vi "Line Configuration Dialog.vi"(8 "error in":errorcluster, 9 "engine configuration in":refnum<class "engine configuration.lvclass">, 10 "tag bus configurable plugin module configuration":refnum<class "SQLite configuration.lvclass">, 11 "Line":T3) -> (0 "error out":errorcluster, 1 "success":bool, 2 "changed":bool, 3 "Mappings out":T2)   [LabVIEW 2014, in "SQLite editor node.lvclass"]
doc: "A dialog for allowing a user to specify the values of a new line."
uses:
  SQLite editor node.lvclass
  module/configuration/Line.ctl
  <vilib>/NI/Tag Bus Module Framework/channel/TBM channel.lvclass
  Mappings.ctl
  Map.ctl
  permissions.ctl
  <vilib>/NI/Module Execution Interface/Engine Configuration/engine configuration.lvclass
  module/configuration/SQLite configuration.lvclass
  <vilib>/NI/Tag Bus Module Framework/channel/TBM channel.lvclass/TBM channel.ctl
  <vilib>/NI/Tag Bus/tag/tag descriptor.lvclass/tag descriptor.ctl
  <vilib>/NI/Configuration Framework/serializable configuration/NISE_CEF_serializable configuration.lvclass/NISE_CEF_serializable configuration.ctl
  <vilib>/NI/Tag Bus/tag/write tag name.vi
  <vilib>/NI/Tag Bus/tag/write data type.vi
  <vilib>/NI/Tag Bus Module Framework/channel/Write channel classification.vi
  <vilib>/NI/Configuration Framework/serializable configuration/Read UID.vi
  <vilib>/NI/Tag Bus Module Framework/channel/Read channel classification.vi
  <vilib>/NI/Tag Bus/tag/read data type.vi
  <vilib>/Utility/LVClass/Get LV Class Name.vi
  <vilib>/NI/Configuration Framework/error generator/NISE_error generator.vi
  <vilib>/NI/Tag Bus/tag/tag descriptor.lvclass
  <vilib>/NI/DCAF UI Toolkit/Controls/DCAF UI Elements.lvlib
panel:
  out "errors":string
  in  "Access Type":T1
  in  "Tag":i32(listbox)
  in  "Data Type":i32(listbox)
  in  "Channel Name":string
  in  "cancel":bool
  in  "ok":bool
  # "#CodeRecommended Add implementation details here. For example, a shared variable URL."
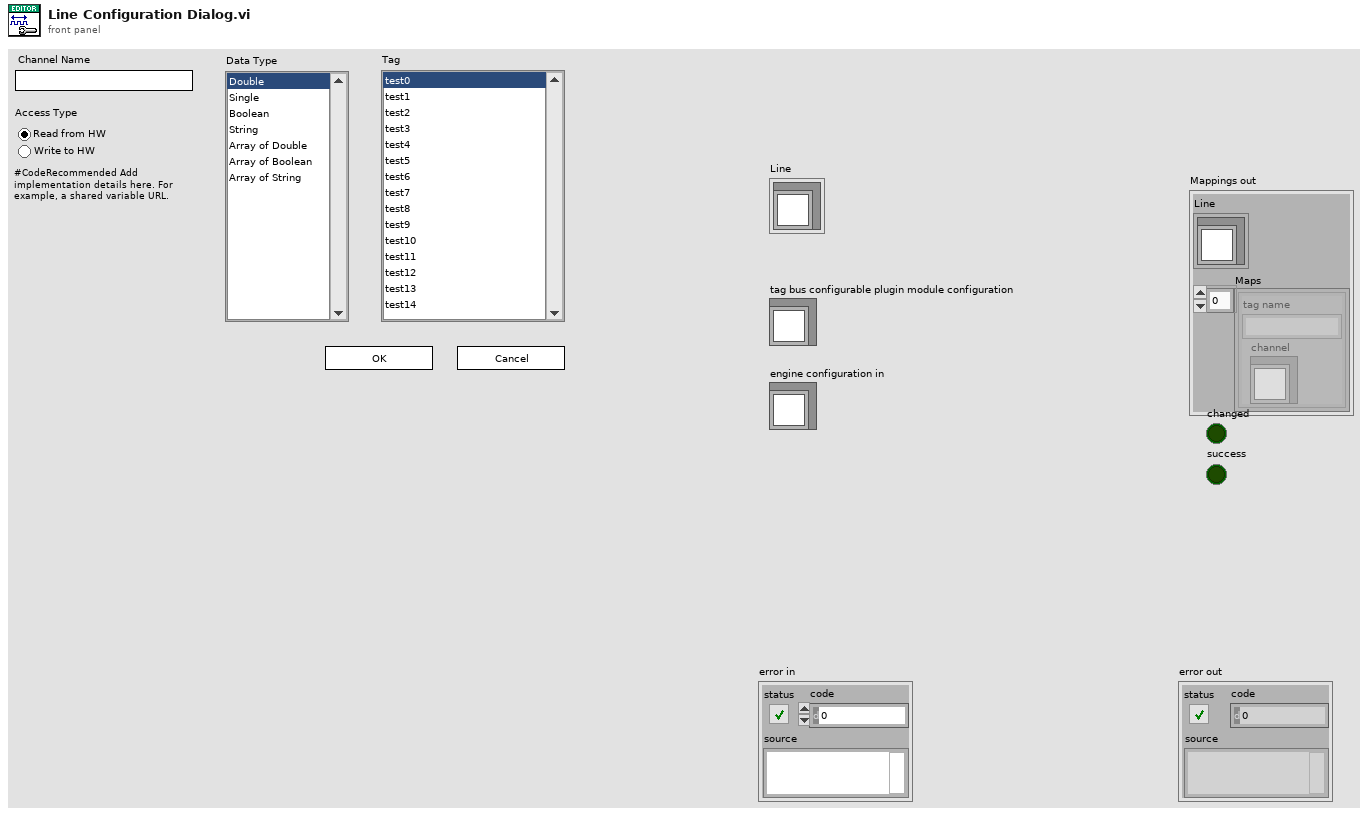
[diagram p1: front panel]
types:
  T1 = typedef "SQLite editor node.lvclass/permissions.ctl" = enum32{"Read from HW", "Write to HW"}
  T2 = typedef "SQLite editor node.lvclass/Mappings.ctl" = cluster{"Line":T3, "Maps":T4[]}
  T3 = typedef "SQLite configuration.lvclass/Line.ctl" = cluster{"channel":refnum<class "TBM channel.lvclass">}
  T4 = typedef "SQLite editor node.lvclass/Map.ctl" = cluster{"channel":refnum<class "TBM channel.lvclass">, "tag name":string}
  T5 = typedef "tag bus.lvlib/tag descriptor.lvclass/Data Type.ctl" = enum16{"Double", "Single", "I64", "I32", "I16", "I8", "U64", "U32", "U16", "U8", "Boolean", "String", "Array of Double", "Array of Single", "Array of I64", "Array of I32", "Array of I16", "Array of I8", "Array of U64", "Array of U32", "Array of U16", "Array of U8", "Array of Boolean", "Array of String"}
  T6 = typedef "TBM channel.lvclass/channel classification.ctl" = enum16{"input data", "output data", "processing parameter", "processing result"}
  T7 = enum8{"Enabled", "Disabled", "Disabled and Grayed Out"}
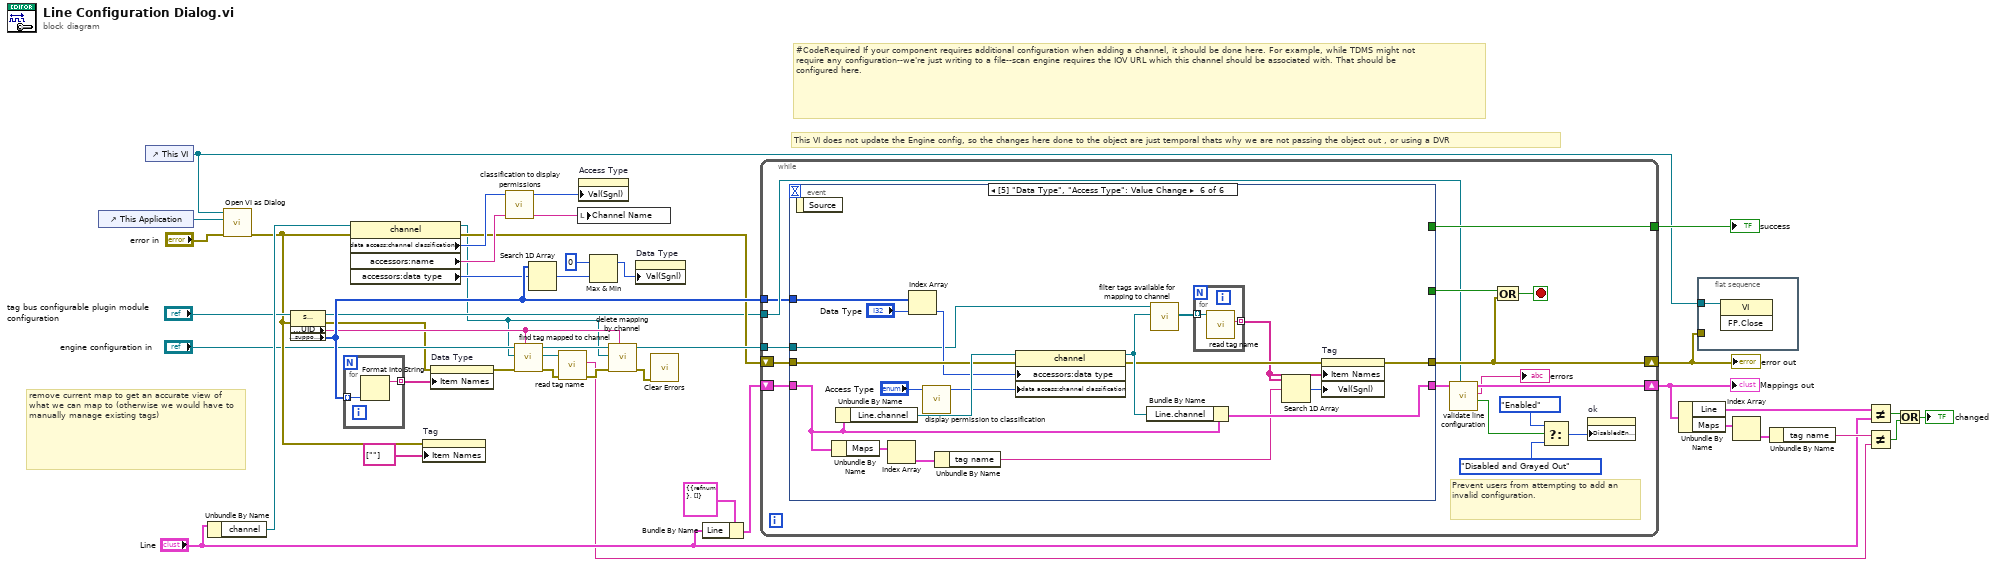
[diagram p0: block diagram]
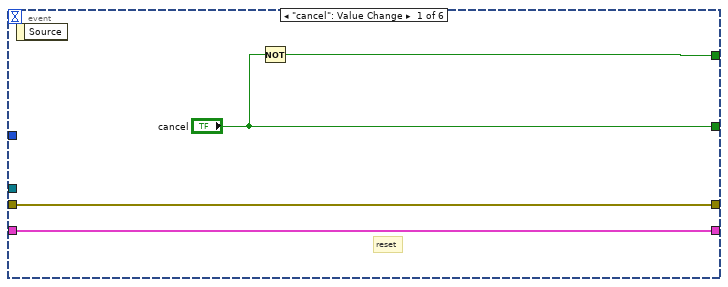
[diagram p2: hidden frame]
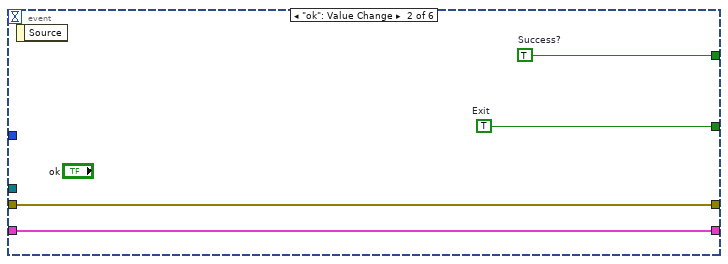
[diagram p3: hidden frame]
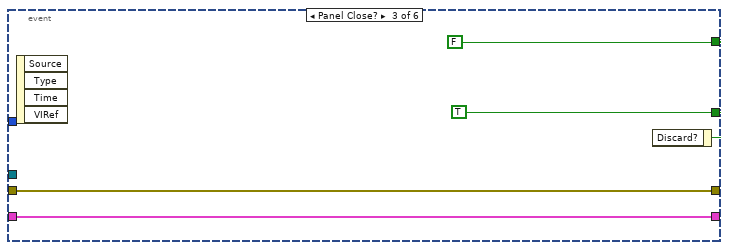
[diagram p4: hidden frame]
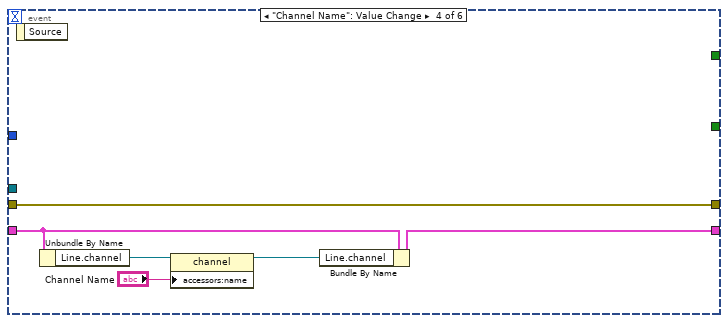
[diagram p5: hidden frame]
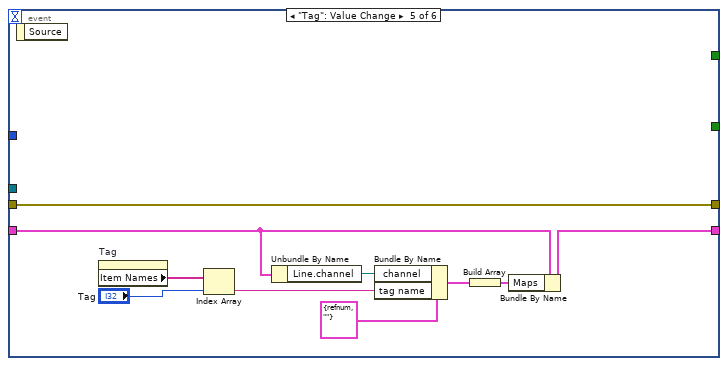
[diagram p6: hidden frame]
diagram:
  # "This VI does not update the Engine config, so the changes here done to the object are just temporal thats why we are not passing the object out , or using a DVR"
  # "remove current map to get an accurate view of what we can map to (otherwise we would have to manually manage existing tags)"
  # "#CodeRequired If your component requires additional configuration when adding a channel, it should be done here. For example, while TDMS might not require any configuration--we're just writing to a file--scan engine requires the IOV URL which this channel should be associated with. That should be configured here."
  n1 = control-ref of="This Application"() -> (w26:refnum<vi>)
  n2 = control-ref of="This VI"() -> (w3:refnum<vi>)
  n3 = Unbundle By Name("Line") -> ("channel"=w37:refnum<class "TBM channel.lvclass">)
  n4 = call <vilib>:"Open VI as Dialog.vi"("error in (no error)"="error in", "This Application"=w26, "VI in"=w3) -> ("error out"=w24:errorcluster)  [unwired: 8 in]
  n5 = property class="SQLite configuration"(reference="tag bus configurable plugin module configuration", error in=w24) -> (reference out=w18:refnum<class "SQLite configuration.lvclass">, error out=w20:errorcluster, "Properties:UID"=w23:string, "Customize:Properties:supported types"=w41:T5[])
  n6 = for {
    tunnel: w41 -> [w45] mode=indexing
    tunnel: [w44] -> w36 mode=indexing
    n7 = Format Into String(w45) -> (resulting string=w44:string)  [unwired: 3 in, 1 out]
  }
  n8 = property class="channel"(reference=w37, error in=w24) -> (reference out=w16:refnum<class "TBM channel.lvclass">, error out=w19:errorcluster, "data access:channel classification"=w39:T6, "accessors:name"=w38:string, "accessors:data type"=w33:T5)
  n9 = property on="Tag" class="LstBox (strict)"(error in=w24, "Item Names"=string[] [""]) -> ()  [unwired: 1 in, 2 out]
  n10 = property on="Data Type" class="LstBox (strict)"(error in=w20, "Item Names"=w36) -> (error out=w17:errorcluster)  [unwired: 1 in, 1 out]
  n11 = call "classification to display permissions.vi"("channel classification"=w39) -> ("permissions"=w34:T1)  [unwired: 10 in]
  n12 = call <vilib>:"find tag mapped to channel.vi"("owner"=w23, "error in"=w17, "channel"=w16, "engine configuration in"="engine configuration in") -> ("error out"=w11:errorcluster, "tag"=w12:refnum<class "tag descriptor.lvclass">, "engine configuration out"=w21:refnum<class "engine configuration.lvclass">)  [unwired: 5 in]
  n13 = Search 1D Array(1D array=w41, element=w33) -> (index of element=w15:i32)  [unwired: 1 in]
  n14 = call <vilib>:"read tag name.vi"("error in"=w11, "system tag in"=w12) -> ("error out"=w10:errorcluster, "name"=w1:string)  [unwired: 7 in, 1 out]
  n15 = local write "Channel Name"(w38) -> ()
  n16 = property on="Access Type" class="RadioBtnsControl (strict)"("Val(Sgnl)"=w34) -> ()  [unwired: 2 in, 2 out]
  n17 = Max & Min(x=0 ("f"), y=w15) -> (max(x,y)=w13:i32)  [unwired: 1 out]
  n18 = call <vilib>:"delete mapping by channel.vi"("owner ID"=w23, "error in"=w10, "channel"=w16, "engine configuration in"=w21) -> ("error out"=w32:errorcluster, "engine configuration out"=w42:refnum<class "engine configuration.lvclass">)  [unwired: 6 in]
  n19 = property on="Data Type" class="LstBox (strict)"("Val(Sgnl)"=w13) -> ()  [unwired: 2 in, 2 out]
  n20 = call <vilib>:"Clear Errors.vi"("error in (no error)"=w32) -> ()  [unwired: 5 in, 2 out]
  n21 = Bundle By Name(cluster=T2 {"Line"={"channel"=refnum}, "Maps"=[]} ("Mappings out"), "Line"="Line") -> (w29:T2)
  n22 = while {
    shift-right: [w53] -> w40
    shift-left: w19 -> [w60]
    tunnel: [w59] -> w43
    shift-right: [w54] -> w27
    shift-left: w29 -> [w56]
    tunnel: w42 -> [w61]
    tunnel: w18 -> [w48]
    tunnel: w41 -> [w47]
    stop <- w57 stop-if-true
    # "Prevent users from attempting to add an invalid configuration."
    n23 = event shown="[5] \"Data Type\", \"Access Type\": Value Change" {
      selector: _ -> [_ _ _ _ _ _]
      dyn-events: _ -> [_ _ _ _ _ _]
      timeout: _ -> [_ _ _ _ _ _]
      tunnel: w61 -> [_ _ _ _ _ w91]
      tunnel: w60 -> [w65 w69 w73 w79 w89 w102]
      tunnel: [w65 w69 w73 w79 w89 w97] -> w53
      tunnel: [w64 w66 FALSE _ _ _] -> w59
      tunnel: ["cancel" w67 w71 _ _ _] -> w58
      tunnel: w56 -> [w62 w68 w70 w77 w84 w90]
      tunnel: [w62 w68 w70 w78 w81 w105] -> w55
      tunnel: w47 -> [_ _ _ _ _ w101]
      event "cancel": Value Change {
        # "reset"
        n24 = event-data() -> ()  [unwired: 1 in, 1 out]
        n25 = Not(x="cancel") -> (.not. x?=w64:bool)
      }
      event "ok": Value Change {
        w66 = TRUE  # Success?
        w67 = TRUE  # Exit
        n26 = event-data() -> ()  [unwired: 1 in, 1 out]
      }
      event Panel Close? {
        w71 = TRUE ("cancel")
        n27 = event-data() -> ()  [unwired: 1 in, 4 out]
        n28 = event-data("Discard?"=w71) -> ()  [unwired: 1 in, 1 out]
      }
      event "Channel Name": Value Change {
        n29 = event-data() -> ()  [unwired: 1 in, 1 out]
        n30 = Unbundle By Name(w77) -> ("Line.channel"=w76:refnum<class "TBM channel.lvclass">)
        n31 = property class="channel"(reference=w76, "accessors:name"="Channel Name") -> (reference out=w75:refnum<class "TBM channel.lvclass">)  [unwired: 1 in, 1 out]
        n32 = Bundle By Name(cluster=w77, "Line.channel"=w75) -> (w78:T2)
      }
      event "Tag": Value Change {
        n33 = event-data() -> ()  [unwired: 1 in, 1 out]
        n34 = property on="Tag" class="LstBox (strict)"() -> ("Item Names"=w87:string[])  [unwired: 2 in, 2 out]
        n35 = Index Array(array=w87, index="Tag") -> (element=w80:string)
        n36 = Unbundle By Name(w84) -> ("Line.channel"=w85:refnum<class "TBM channel.lvclass">)
        n37 = Bundle By Name(cluster=T4 {"channel"=refnum, "tag name"=""} ("Map"), "channel"=w85, "tag name"=w80) -> (w83:T4)
        n38 = Build Array(w83) -> (w82:T4[])
        n39 = Bundle By Name(cluster=w84, "Maps"=w82) -> (w81:T2)
      }
      event "Data Type": Value Change {
        n40 = event-data() -> ()  [unwired: 1 in, 1 out]
        n41 = Unbundle By Name(w90) -> ("Maps"=w94:T4[])
        n42 = Unbundle By Name(w90) -> ("Line.channel"=w108:refnum<class "TBM channel.lvclass">)
        n43 = Index Array(array=w94) -> (element=w93:T4)  [unwired: 1 in]
        n44 = Index Array(array=w101, index="Data Type") -> (element=w99:T5)
        n45 = call "display permission to classification.vi"("display permissions"="Access Type") -> ("channel classification"=w107:T6)  [unwired: 10 in]
        n46 = Unbundle By Name(w93) -> ("tag name"=w92:string)
        n47 = property class="channel"(reference=w108, error in=w102, "accessors:data type"=w99, "data access:channel classification"=w107) -> (reference out=w106:refnum<class "TBM channel.lvclass">, error out=w98:errorcluster)
        n48 = Bundle By Name(cluster=w90, "Line.channel"=w106) -> (w105:T2)
        n49 = call-dynamic "filter tags available for mapping to channel.vi"("channel to map to"=w106, "engine configuration in"=w91) -> ("filtered tags"=w104:refnum<class "tag descriptor.lvclass">[])  [unwired: 8 in, 1 out]
        n50 = for {
          tunnel: w104 -> [w110] mode=indexing
          tunnel: [w109] -> w96 mode=indexing
          n51 = call <vilib>:"read tag name.vi"("system tag in"=w110) -> ("name"=w109:string)  [unwired: 8 in, 2 out]
        }
        n52 = Search 1D Array(1D array=w96, element=w92) -> (index of element=w95:i32)  [unwired: 1 in]
        n53 = property on="Tag" class="LstBox (strict)"(error in=w98, "Item Names"=w96, "Val(Sgnl)"=w95) -> (error out=w97:errorcluster)  [unwired: 1 in, 1 out]
      }
    }
    n54 = call "validate line configuration.vi"("Module Config"=w48, "Mappings in"=w55) -> ("valid?"=w52:bool, "errors"=→"errors":string, "Mappings out"=w54:T2)  [unwired: 7 in]
    n55 = Compound Arithmetic op=OR(w58, w53) -> (w57:bool)
    n56 = Select(t=T7."Enabled" ("Disabled"), s=w52, f=T7."Disabled and Grayed Out") -> (s? t:f=w49:T7)
    n57 = property on="ok" class="Bool"("DisabledEnum"=w49) -> ()  [unwired: 2 in, 2 out]
  }
  "error out" <- w40
  "success" <- w43
  "Mappings out" <- w27
  n58 = Unbundle By Name(w27) -> ("Line"=w28:T3, "Maps"=w9:T4[])
  n59 = flat-sequence {
    tunnel: w40 -> [_]
    tunnel: w3 -> [w111]
    frame #0 {
      n60 = invoke class="VI" method="FP.Close"(reference=w111) -> ()  [unwired: 2 in, 3 out]
    }
  }
  n61 = Index Array(array=w9) -> (element=w8:T4)  [unwired: 1 in]
  n62 = Unbundle By Name(w8) -> ("tag name"=w7:string)
  n63 = Not Equal?(x=w28, y="Line") -> (x != y?=w5:bool)
  n64 = Not Equal?(x=w7, y=w1) -> (x != y?=w6:bool)
  n65 = Or(x=w5, y=w6) -> (x .or. y?=→"changed":bool)
